vi "Write Theme File Path.vi"(8 "error in (no error)":errorcluster, 10 "Theme File Path":path, 11 "Appearance Actor in":refnum<class "Appearance Actor.lvclass">) -> (0 "error out":errorcluster, 3 "Appearance Actor out":refnum<class "Appearance Actor.lvclass">)   [LabVIEW 2021, in "Appearance Actor.lvlib" / "Appearance Actor.lvclass"]
uses:
  Appearance Actor.lvclass
  Appearance Actor.lvclass/Appearance Actor.ctl
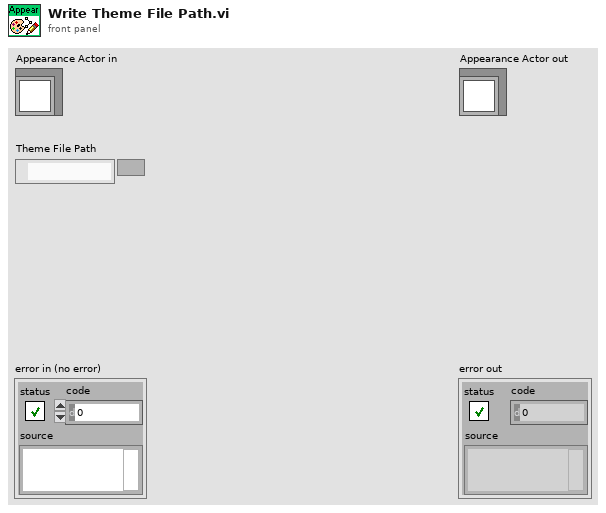
[diagram p1: front panel]
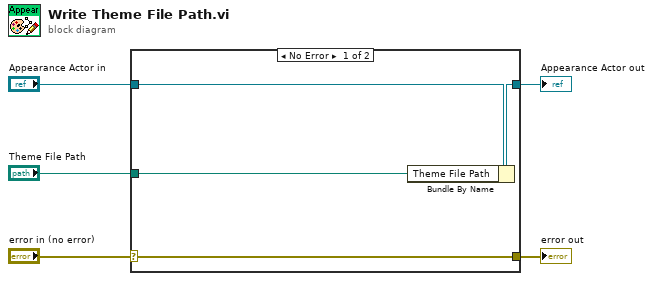
[diagram p0: block diagram]
diagram:
  n1 = case shown="No Error" "error in (no error)" {
    selector: "error in (no error)" -> [w9 w10]
    tunnel: [w9 w10] -> w4
    tunnel: [w7 w11] -> w2
    tunnel: "Appearance Actor in" -> [w8 w11]
    tunnel: "Theme File Path" -> [w6 _]
    frame No Error {
      n2 = Bundle By Name(cluster=w8, "Theme File Path"=w6) -> (w7:refnum<class "Appearance Actor.lvclass">)
    }
    frame Error {
    }
  }
  "error out" <- w4
  "Appearance Actor out" <- w2
